vi "SSH Putty.vi"(8 "error in":errorcluster, 9 "Command(s) to Execute":string="cd /", 11 "Password":string="Hotel2planet!*#)") -> (0 "error out":errorcluster, 1 "std error":string, 3 "std output":string)   [LabVIEW 2021]
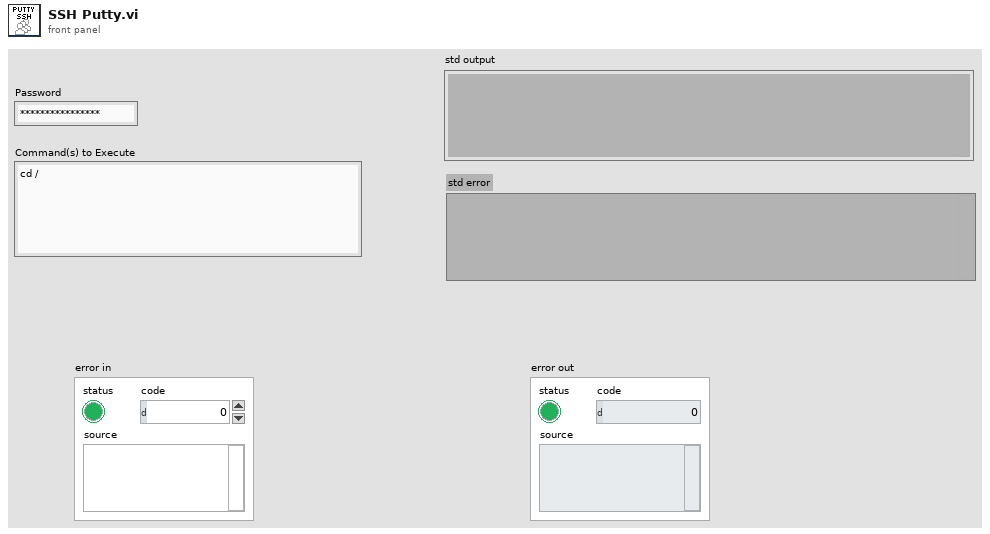
[diagram p1: front panel]
types:
  T1 = enum16{"open", "replace", "create", "open or create", "replace or create", "replace or create with confirmation"}
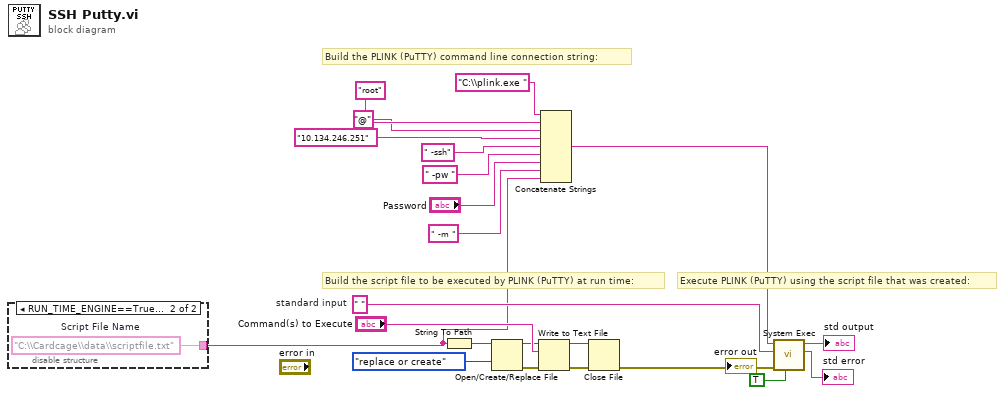
[diagram p0: block diagram]
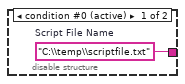
[diagram p2: hidden frame]
diagram:
  w14 = " "  # standard input
  # "Execute PLINK (PuTTY) using the script file that was created:"
  # "Build the script file to be executed by PLINK (PuTTY) at run time:"
  # "Build the PLINK (PuTTY) command line connection string:"
  n1 = disable-structure "Conditional Disable Structure" shown="RUN_TIME_ENGINE==True&&OS==Win" {
    disable-tunnel: [w23 w24] -> w1
    frame condition #0 (active) {
      w23 = "C:\\temp\\scriptfile.txt"  # Script File Name
    }
    frame condition #1 {
      w24 = "C:\\Cardcage\\data\\scriptfile.txt"  # Script File Name
    }
  }
  n2 = String To Path(string=w1) -> (path=w4:path)
  n3 = Open/Create/Replace File(file path (use dialog)=w4, operation (0:open)=T1."replace or create") -> (refnum out=w17:refnum<file>, error out=w16:errorcluster)  [unwired: 4 in, 1 out]
  n4 = Write to Text File(file (use dialog)=w17, text="Command(s) to Execute", error in=w16) -> (refnum out=w20:refnum<file>, error out=w19:errorcluster)  [unwired: 2 out]
  n5 = Concatenate Strings("C:\\plink.exe " ("command line"), "root" ("Username"), "@" ("string"), "10.134.246.251" ("Host"), " -ssh", " -pw " ("string"), "Password", " -m " ("string"), w1) -> (w5:string)
  n6 = Close File(refnum=w20, error in=w19) -> (error out=w18:errorcluster)  [unwired: 1 out]
  n7 = call <vilib>:"System Exec.vi"("run minimized? (F)"=TRUE, "error in (no error)"=w18, "standard input"=w14, "command line"=w5) -> ("standard error"=→"std error":string, "standard output"=→"std output":string)  [unwired: 2 in, 4 out]
